vi "Read Global Position.vi"(8 "error in (no error)":errorcluster, 11 "DFRobot_Gravity_GNSS in":refnum<class "DFRobot_Gravity_GNSS.lvclass">) -> (0 "error out":errorcluster, 1 "string":string, 2 "GPSReturn":T1 {"UTC Time Stamp" format="%<%.3X>T"; "Longitude" format="%#_12f"; "Latitude" format="%#_12f"}, 3 "DFRobot_Gravity_GNSS out":refnum<class "DFRobot_Gravity_GNSS.lvclass">)   [LabVIEW 2020, in "CTI-Peripheral.lvlib" / "DFRobot_Gravity_GNSS.lvclass"]
uses:
  DFRobot_Gravity_GNSS.lvclass
  DFRobot_Gravity_GNSS.lvclass/DFRobot_Gravity_GNSS.ctl
  CTI/I2C Connection/I2C Connection.lvclass
  Private/GPSData.ctl
  96fe237b-d73c-496c-bb0d-b127a2e84b77.vi
  Private/GPSReturn.ctl
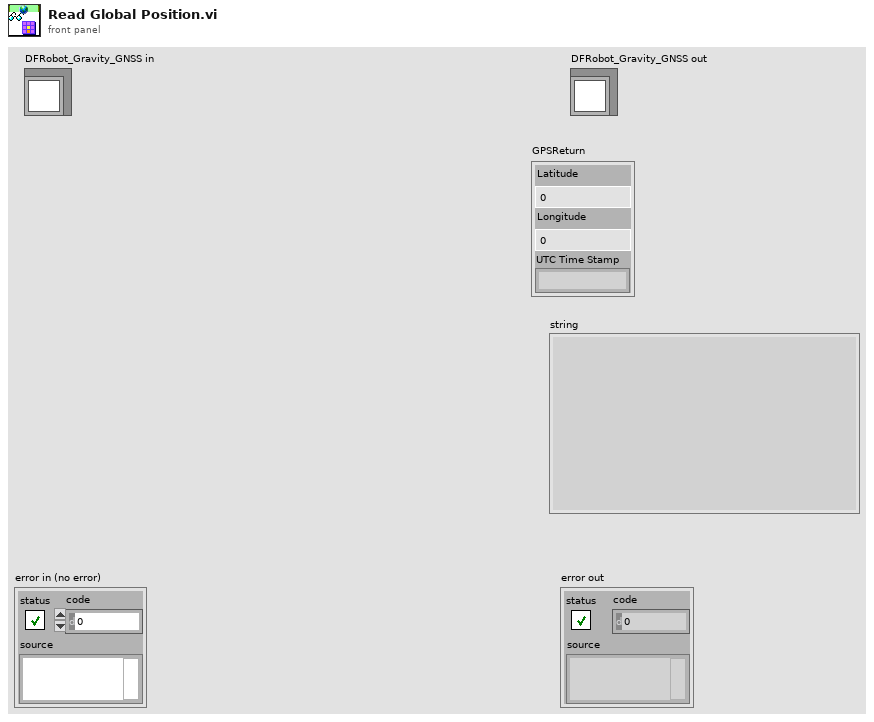
[diagram p1: front panel]
types:
  T1 = typedef "CTI-Peripheral.lvlib/DFRobot_Gravity_GNSS.lvclass/GPSReturn.ctl" = cluster{"Latitude":dbl, "Longitude":dbl, "UTC Time Stamp":timestamp}
  T2 = typedef "CTI-Peripheral.lvlib/DFRobot_Gravity_GNSS.lvclass/GPSData.ctl" = u16
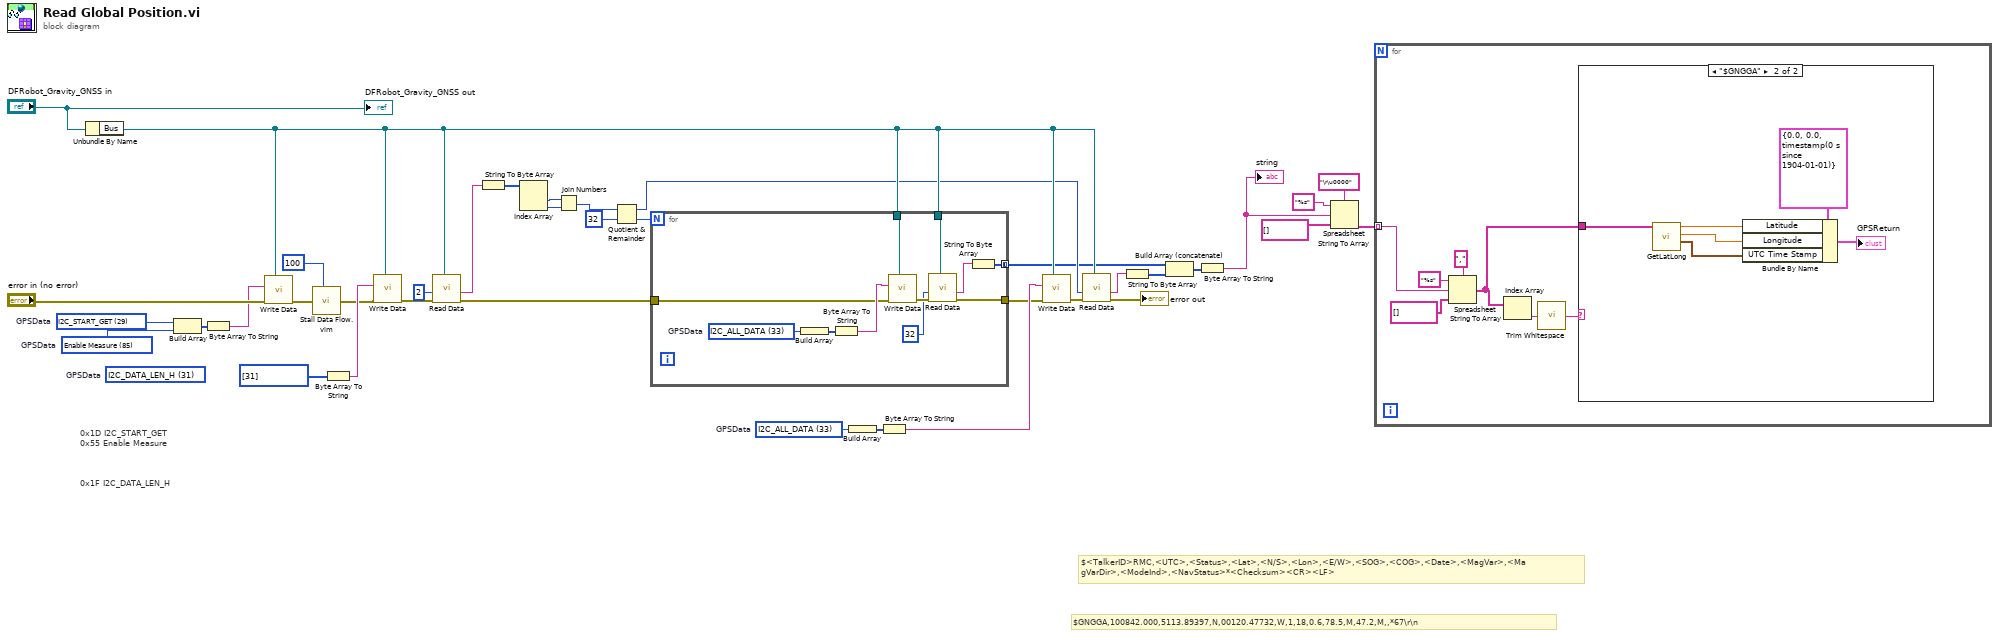
[diagram p0: block diagram]
diagram:
  w17 = T2 33 items=["I2C_YEAR_H", "I2C_YEAR_L", "I2C_MONTH", "I2C_DATE", "I2C_HOUR", "I2C_MINUTE", "I2C_SECOND", "I2C_LAT_1", "I2C_LAT_2", "I2C_LAT_X_24", "I2C_LAT_X_16", "I2C_LAT_X_8", "I2C_LON_DIS", "I2C_LON_1", "I2C_LON_2", "I2C_LON_X_24", "I2C_LON_X_16", "I2C_LON_X_8", "I2C_LAT_DIS", "I2C_USE_STAR", "I2C_ALT_H", "I2C_ALT_L", "I2C_ALT_X", "I2C_SOG_H", "I2C_SOG_L", "I2C_SOG_X", "I2C_COG_H", "I2C_COG_L", "I2C_COG_X", "I2C_START_GET", "I2C_ID", "I2C_DATA_LEN_H", "I2C_DATA_LEN_L", "I2C_ALL_DATA", "I2C_GNSS_MODE", "I2C_SLEEP_MODE", "I2C_RGB_MODE"]  # GPSData
  (unwired) T2 31 items=["I2C_YEAR_H", "I2C_YEAR_L", "I2C_MONTH", "I2C_DATE", "I2C_HOUR", "I2C_MINUTE", "I2C_SECOND", "I2C_LAT_1", "I2C_LAT_2", "I2C_LAT_X_24", "I2C_LAT_X_16", "I2C_LAT_X_8", "I2C_LON_DIS", "I2C_LON_1", "I2C_LON_2", "I2C_LON_X_24", "I2C_LON_X_16", "I2C_LON_X_8", "I2C_LAT_DIS", "I2C_USE_STAR", "I2C_ALT_H", "I2C_ALT_L", "I2C_ALT_X", "I2C_SOG_H", "I2C_SOG_L", "I2C_SOG_X", "I2C_COG_H", "I2C_COG_L", "I2C_COG_X", "I2C_START_GET", "I2C_ID", "I2C_DATA_LEN_H", "I2C_DATA_LEN_L", "I2C_ALL_DATA", "I2C_GNSS_MODE", "I2C_SLEEP_MODE", "I2C_RGB_MODE"]  # GPSData
  w34 = T2 85 items=["I2C_YEAR_H"=0, "I2C_YEAR_L"=1, "I2C_MONTH"=2, "I2C_DATE"=3, "I2C_HOUR"=4, "I2C_MINUTE"=5, "I2C_SECOND"=6, "I2C_LAT_1"=7, "I2C_LAT_2"=8, "I2C_LAT_X_24"=9, "I2C_LAT_X_16"=10, "I2C_LAT_X_8"=11, "I2C_LON_DIS"=12, "I2C_LON_1"=13, "I2C_LON_2"=14, "I2C_LON_X_24"=15, "I2C_LON_X_16"=16, "I2C_LON_X_8"=17, "I2C_LAT_DIS"=18, "I2C_USE_STAR"=19, "I2C_ALT_H"=20, "I2C_ALT_L"=21, "I2C_ALT_X"=22, "I2C_SOG_H"=23, "I2C_SOG_L"=24, "I2C_SOG_X"=25, "I2C_COG_H"=26, "I2C_COG_L"=27, "I2C_COG_X"=28, "I2C_START_GET"=29, "I2C_ID"=30, "I2C_DATA_LEN_H"=31, "I2C_DATA_LEN_L"=32, "I2C_ALL_DATA"=33, "I2C_GNSS_MODE"=34, "I2C_SLEEP_MODE"=35, "I2C_RGB_MODE"=36, "Enable Measure"=85]  # GPSData
  w35 = T2 29 items=["I2C_YEAR_H", "I2C_YEAR_L", "I2C_MONTH", "I2C_DATE", "I2C_HOUR", "I2C_MINUTE", "I2C_SECOND", "I2C_LAT_1", "I2C_LAT_2", "I2C_LAT_X_24", "I2C_LAT_X_16", "I2C_LAT_X_8", "I2C_LON_DIS", "I2C_LON_1", "I2C_LON_2", "I2C_LON_X_24", "I2C_LON_X_16", "I2C_LON_X_8", "I2C_LAT_DIS", "I2C_USE_STAR", "I2C_ALT_H", "I2C_ALT_L", "I2C_ALT_X", "I2C_SOG_H", "I2C_SOG_L", "I2C_SOG_X", "I2C_COG_H", "I2C_COG_L", "I2C_COG_X", "I2C_START_GET", "I2C_ID", "I2C_DATA_LEN_H", "I2C_DATA_LEN_L", "I2C_ALL_DATA", "I2C_GNSS_MODE", "I2C_SLEEP_MODE", "I2C_RGB_MODE"]  # GPSData
  # "0x1D\tI2C_START_GET \n0x55\tEnable Measure\n\t\n\t\n\t\n0x1F\tI2C_DATA_LEN_H"
  # "$GNGGA,100842.000,5113.89397,N,00120.47732,W,1,18,0.6,78.5,M,47.2,M,,*67\\r\\n"
  # "$<TalkerID>RMC,<UTC>,<Status>,<Lat>,<N/S>,<Lon>,<E/W>,<SOG>,<COG>,<Date>,<MagVar>,<Ma\ngVarDir>,<ModeInd>,<NavStatus>*<Checksum><CR><LF>"
  n1 = Unbundle By Name("DFRobot_Gravity_GNSS in") -> ("Bus"=w11:refnum<class "I2C Connection.lvclass">)
  n2 = Build Array(w35, w34) -> (w36:T2[])
  n3 = Byte Array To String(unsigned byte array=w36) -> (string=w33:string)
  n4 = call "Write Data.vi"("I2C Connection"=w11, "error in (no error)"="error in (no error)", "Data"=w33) -> ("error out"=w32:errorcluster)  [unwired: 8 in]
  n5 = call "Stall Data Flow.vim"("value in"=w32, "milliseconds to wait"=u32 100) -> ("value out"=w22:errorcluster)  [unwired: 1 out]
  n6 = Byte Array To String(unsigned byte array=u8[] [31]) -> (string=w31:string)
  n7 = call "Write Data.vi"("I2C Connection"=w11, "error in (no error)"=w22, "Data"=w31) -> ("error out"=w30:errorcluster)  [unwired: 8 in]
  n8 = call "Read Data.vi"("I2C Connection"=w11, "error in (no error)"=w30, "Len"=u8 2) -> ("error out"=w28:errorcluster, "Data"=w27:string)  [unwired: 7 in]
  n9 = String To Byte Array(string=w27) -> (unsigned byte array=w26:u8[])
  n10 = Index Array(array=w26) -> (element #1=w24:u8, element #2=w25:u8)  [unwired: 2 in]
  n11 = Join Numbers(hi=w24, lo=w25) -> ((hi.lo)=w20:u16)
  n12 = Quotient & Remainder(x=w20, y=u16 32) -> (x-y*floor(x/y)=w10:u16, floor(x/y)=w18:u16)
  n13 = for {
    N: w18 -> [_]
    tunnel: [w48] -> w8 mode=concatenating
    tunnel: w28 -> [w45]
    tunnel: [w43] -> w12
    tunnel: w11 -> [w42]
    tunnel: w11 -> [w41]
    w39 = T2 33 items=["I2C_YEAR_H", "I2C_YEAR_L", "I2C_MONTH", "I2C_DATE", "I2C_HOUR", "I2C_MINUTE", "I2C_SECOND", "I2C_LAT_1", "I2C_LAT_2", "I2C_LAT_X_24", "I2C_LAT_X_16", "I2C_LAT_X_8", "I2C_LON_DIS", "I2C_LON_1", "I2C_LON_2", "I2C_LON_X_24", "I2C_LON_X_16", "I2C_LON_X_8", "I2C_LAT_DIS", "I2C_USE_STAR", "I2C_ALT_H", "I2C_ALT_L", "I2C_ALT_X", "I2C_SOG_H", "I2C_SOG_L", "I2C_SOG_X", "I2C_COG_H", "I2C_COG_L", "I2C_COG_X", "I2C_START_GET", "I2C_ID", "I2C_DATA_LEN_H", "I2C_DATA_LEN_L", "I2C_ALL_DATA", "I2C_GNSS_MODE", "I2C_SLEEP_MODE", "I2C_RGB_MODE"]  # GPSData
    n14 = Build Array(w39) -> (w49:T2[])
    n15 = Byte Array To String(unsigned byte array=w49) -> (string=w47:string)
    n16 = call "Write Data.vi"("I2C Connection"=w42, "error in (no error)"=w45, "Data"=w47) -> ("error out"=w46:errorcluster)  [unwired: 8 in]
    n17 = call "Read Data.vi"("I2C Connection"=w41, "error in (no error)"=w46, "Len"=u8 32) -> ("error out"=w43:errorcluster, "Data"=w44:string)  [unwired: 7 in]
    n18 = String To Byte Array(string=w44) -> (unsigned byte array=w48:u8[])
  }
  n19 = Build Array(w17) -> (w13:T2[])
  n20 = Byte Array To String(unsigned byte array=w13) -> (string=w14:string)
  n21 = call "Write Data.vi"("I2C Connection"=w11, "error in (no error)"=w12, "Data"=w14) -> ("error out"=w15:errorcluster)  [unwired: 8 in]
  n22 = call "Read Data.vi"("I2C Connection"=w11, "error in (no error)"=w15, "Len"=w10) -> ("error out"=→"error out":errorcluster, "Data"=w16:string)  [unwired: 7 in]
  n23 = String To Byte Array(string=w16) -> (unsigned byte array=w9:u8[])
  n24 = Build Array (concatenate)(w8, w9) -> (w7:u8[])
  n25 = Byte Array To String(unsigned byte array=w7) -> (string=w3:string)
  "string" <- w3
  n26 = Spreadsheet String To Array(delimiter (Tab)="\r\u0000" ("format string"), format string="%s", spreadsheet string=w3, array type (2D Dbl)=string[] []) -> (array=w2:string[])
  n27 = for {
    tunnel: w2 -> [w53] mode=indexing
    n28 = Spreadsheet String To Array(delimiter (Tab)=",", format string="%s", spreadsheet string=w53, array type (2D Dbl)=string[] []) -> (array=w52:string[])
    n29 = Index Array(array=w52) -> (element=w51:string)  [unwired: 1 in]
    n30 = call <vilib>:"Trim Whitespace.vi"("string"=w51) -> ("trimmed string"=w50:string)  [unwired: 1 in]
    n31 = case shown="\"$GNGGA\"" w50 {
      tunnel: w52 -> [_ w57]
      frame "False", Default {
      }
      frame "$GNGGA" {
        n32 = call "GetLatLong.vi"("Fields"=w57) -> ("UTC Time Stamp"=w58:timestamp, "Longitude"=w59:dbl, "Latitude"=w61:dbl)  [unwired: 8 in]
        n33 = Bundle By Name(cluster=T1 {"Latitude"=0.0, "Longitude"=0.0, "UTC Time Stamp"=timestamp(0 s since 1904-01-01)} ("GPSReturn"), "Latitude"=w61, "Longitude"=w59, "UTC Time Stamp"=w58) -> (→"GPSReturn":T1)
      }
    }
  }
  "DFRobot_Gravity_GNSS out" <- "DFRobot_Gravity_GNSS in"
